vi "Run Tests.vi"() -> ()   [LabVIEW 2020]
panel:
  out "Array":cluster{string, bool}[](array[cluster])
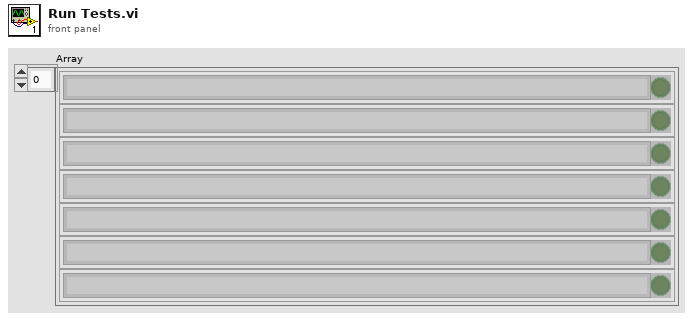
[diagram p1: front panel]
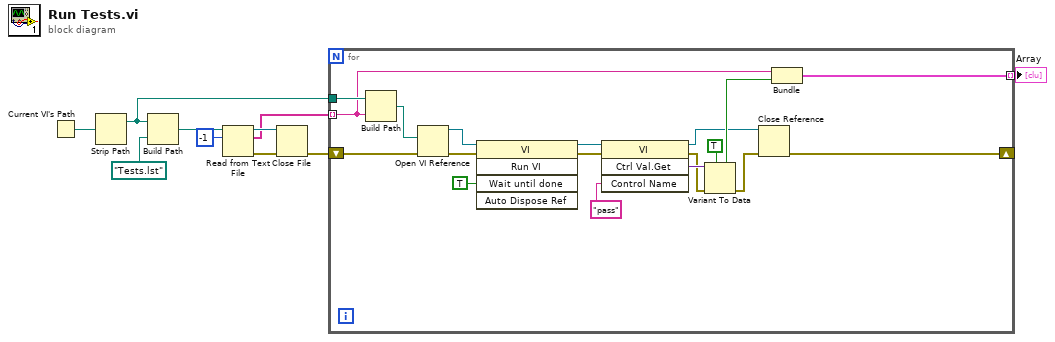
[diagram p0: block diagram]
diagram:
  n1 = Current VI's Path() -> (path=w10:path)
  n2 = Strip Path(path=w10) -> (stripped path=w2:path)  [unwired: 1 out]
  n3 = Build Path(base path=w2, name or relative path=path "Tests.lst" ("file (use dialog)")) -> (appended path=w8:path)
  n4 = Read from Text File(file (use dialog)=w8, count=-1) -> (refnum out=w6:refnum<file>, text=w4:string[], error out=w7:errorcluster)  [unwired: 2 in, 1 out]
  n5 = Close File(refnum=w6, error in=w7) -> (error out=w5:errorcluster)  [unwired: 1 out]
  n6 = for {
    shift-right: [w11] -> _
    shift-left: w5 -> [w27]
    tunnel: w4 -> [w16] mode=indexing
    tunnel: w2 -> [w28]
    tunnel: [w14] -> w1 mode=indexing
    n7 = Build Path(base path=w28, name or relative path=w16) -> (appended path=w26:path)
    n8 = Open VI Reference(vi path=w26, error in (no error)=w27) -> (vi reference=w25:refnum<vi>, error out=w24:errorcluster)  [unwired: 4 in]
    n9 = invoke class="VI" method="Run VI"(reference=w25, error in=w24, "Wait until done"=TRUE ("Wait Until Done")) -> (reference out=w22:refnum<vi>, error out=w21:errorcluster)  [unwired: 2 in, 3 out]
    n10 = invoke class="VI" method="Ctrl Val.Get"(reference=w22, error in=w21, "Control Name"="pass") -> (reference out=w13:refnum<vi>, error out=w18:errorcluster, "Get Control Value Variant"=w19:variant)  [unwired: 1 in, 1 out]
    n11 = Variant To Data(error in=w18, type=TRUE, Variant=w19) -> (data=w15:bool, error out=w12:errorcluster)
    n12 = Close Reference(reference=w13, error in (no error)=w12) -> (error out=w11:errorcluster)
    n13 = Bundle(w16, w15) -> (w14:cluster{string, bool})  [unwired: 1 in]
  }
  "Array" <- w1
